vi "e.gate HighSpeedPort Query.vi"(0 "TCP-Connection (Refnum in)":refnum<k5>, 5 "Command (In)":string, 7 "Timeout":i32, 9 "TCP LengthRead":i32, 11 "error in (no error)":errorcluster) -> (4 "TCP-Connection (Refnum out)":refnum<k5>, 6 "Data (out - binary)":u8[](array[numeric]), 8 "data out (string)":string, 15 "error out":errorcluster)   [LabVIEW 2016]
doc: "This VI is used for data transfer over HighSpeedPort TCP/IP."
panel:
  out "Daten":string
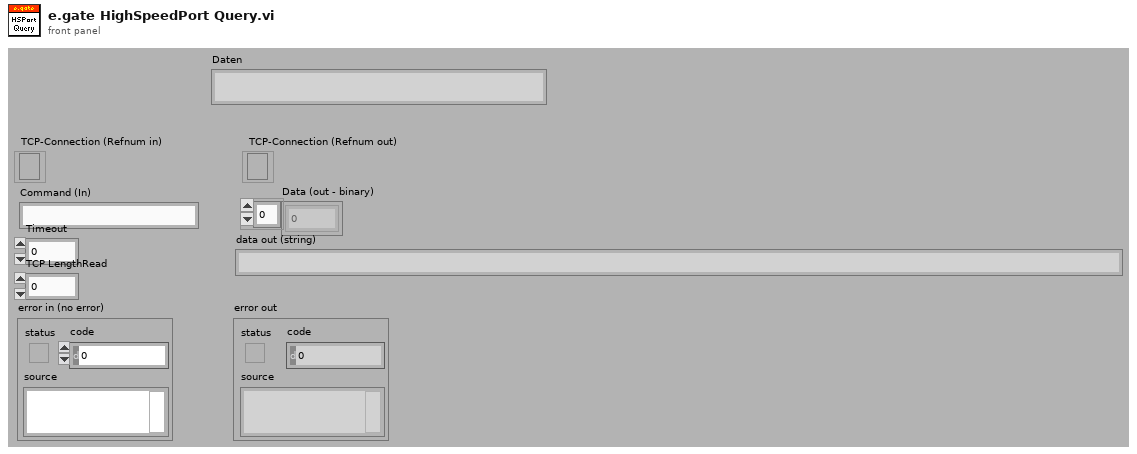
[diagram p1: front panel]
types:
  T1 = enum16{"Standard", "Buffered", "CRLF", "Immediate"}
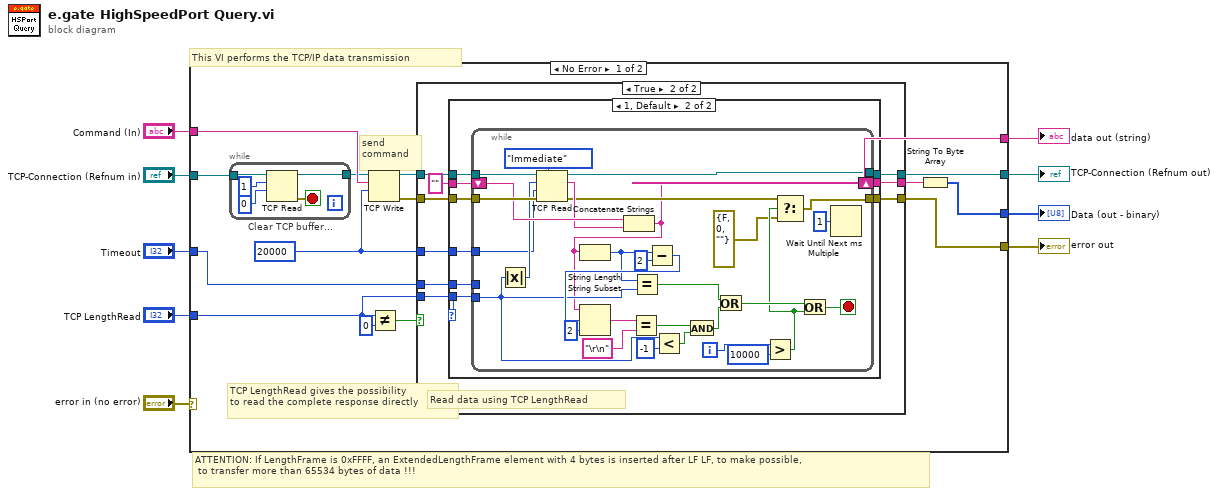
[diagram p0: block diagram]
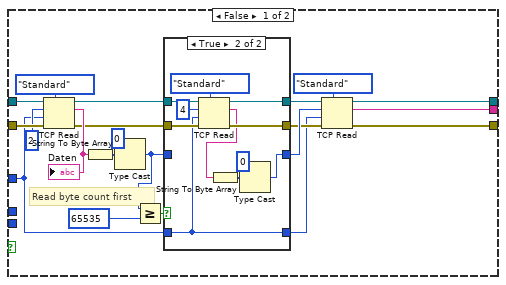
[diagram p2: hidden frame]
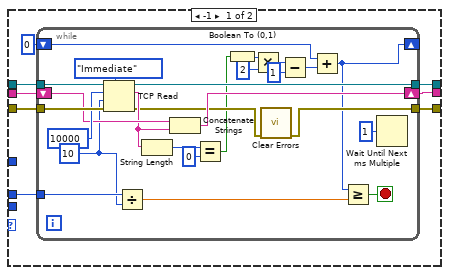
[diagram p4: hidden frame]
diagram:
  # "ATTENTION: If LengthFrame is 0xFFFF, an ExtendedLengthFrame element with 4 bytes is inserted after LF LF, to make possible,\n\tto transfer more than 65534 bytes of data !!!"
  # "This VI performs the TCP/IP data transmission"
  n1 = case shown="No Error" "error in (no error)" {
    selector: "error in (no error)" -> [_ w146]
    tunnel: "TCP-Connection (Refnum in)" -> [w20 w147]
    tunnel: "Timeout" -> [w11 _]
    tunnel: [w23 w147] -> w7
    tunnel: [w22 w146] -> w1
    tunnel: [w21 _] -> w6
    tunnel: "TCP LengthRead" -> [w19 _]
    tunnel: [w18 _] -> w4
    tunnel: "Command (In)" -> [w17 _]
    frame No Error {
      w10 = 20000 ("Timeout")
      # "TCP LengthRead gives the possibility\nto read the complete response directly"
      # "send\ncommand"
      n2 = while "Clear TCP buffer..." {
        tunnel: [w144] -> w14
        tunnel: w20 -> [w141]
        stop <- w145 stop-if-true
        n3 = TCP Read(connection ID=w141, bytes to read=1, 9:0 ("Timeout in ms (25000)")) -> (connection ID out=w144:refnum<k5>, error out=w145:errorcluster)  [unwired: 1 in, 2 out]
      }
      n4 = TCP Write ("TCP: Schreiben")(connection ID=w14, data in=w17, 9:w10) -> (connection ID out=w15:refnum<k5>, error out=w16:errorcluster)  [unwired: 1 in, 1 out]
      n5 = Not Equal?(x=w19, y=0) -> (x != y?=w12:bool)
      n6 = case shown="True" w12 {
        tunnel: w16 -> [w44 w67]
        tunnel: w15 -> [w43 w68]
        tunnel: [w36 w65] -> w23
        tunnel: [w35 w66] -> w22
        tunnel: [w34 w64] -> w18
        tunnel: w10 -> [w25 w63]
        tunnel: w19 -> [_ w60]
        tunnel: w11 -> [_ w61]
        frame False {
          # "Read byte count first"
          n7 = TCP Read ("TCP: Lesen")(connection ID=w43, bytes to read=2 ("Bytes zu lesen"), error in (no error)=w44, 7:T1."Standard" ("Modus (Standard)"), 9:w25) -> (connection ID out=w30:refnum<k5>, data out=w38:string, error out=w32:errorcluster)
          "Daten" <- w38
          n8 = String To Byte Array(string=w38) -> (unsigned byte array=w39:u8[])
          n9 = Type Cast(type=u16 0, x=w39) -> (*(type *) &x=w27:u16)
          n10 = Greater Or Equal?(x=w27, y=65535) -> (x >= y?=w28:bool)
          n11 = case shown="True" w28 {
            tunnel: w27 -> [w48 _]
            tunnel: [w48 w49] -> w33
            tunnel: w32 -> [w47 w56]
            tunnel: [w47 w55] -> w31
            tunnel: w30 -> [w46 w57]
            tunnel: [w46 w58] -> w29
            tunnel: w25 -> [w45 w54]
            tunnel: [w45 w54] -> w24
            frame False {
            }
            frame True {
              n12 = TCP Read ("TCP: Lesen")(connection ID=w57, bytes to read=4 ("Bytes zu lesen"), error in (no error)=w56, 7:T1."Standard" ("Modus (Standard)"), 9:w54) -> (connection ID out=w58:refnum<k5>, data out=w50:string, error out=w55:errorcluster)
              n13 = String To Byte Array(string=w50) -> (unsigned byte array=w52:u8[])
              n14 = Type Cast(type=u32 0, x=w52) -> (*(type *) &x=w49:u32)
            }
          }
          n15 = TCP Read ("TCP: Lesen")(connection ID=w29, bytes to read=w33, error in (no error)=w31, 7:T1."Standard" ("Modus (Standard)"), 9:w24) -> (connection ID out=w36:refnum<k5>, data out=w34:string, error out=w35:errorcluster)
        }
        frame True {
          # "Read data using TCP LengthRead"
          n16 = case shown="1, Default" w60 {
            tunnel: w68 -> [w73 w110]
            tunnel: w67 -> [w71 w109]
            tunnel: [w74 w108] -> w66
            tunnel: [w75 w107] -> w65
            tunnel: [w76 w106] -> w64
            tunnel: w63 -> [_ w105]
            tunnel: w60 -> [_ w104]
            tunnel: "" -> [w72 w103]
            tunnel: w61 -> [w70 w102]
            frame -1 {
              n17 = while {
                tunnel: w73 -> [w101]
                tunnel: [w99] -> w75
                shift-right: [w94] -> w76
                shift-left: w72 -> [w95]
                tunnel: w71 -> [w100]
                tunnel: [w85] -> w74
                tunnel: w70 -> [w90]
                shift-right: [w77] -> _
                shift-left: 0 ("y") -> [w91]
                stop <- w87 stop-if-true
                w89 = 10 ("Timeout in ms (25000)")
                n18 = TCP Read(connection ID=w101, bytes to read=10000 ("Bytes zu lesen"), error in (no error)=w100, 7:T1."Immediate" ("Modus (Standard)"), 9:w89) -> (connection ID out=w99:refnum<k5>, data out=w92:string, error out=w86:errorcluster)
                n19 = Divide(x=w90, y=w89) -> (x/y=w88:dbl)
                n20 = String Length(string=w92) -> (length=w84:i32)
                n21 = Concatenate Strings(w95, w92) -> (w94:string)
                n22 = Equal?(x=w84, y=0) -> (x = y?=w83:bool)
                n23 = Boolean To (0,1)(Boolean=w83) -> (0, 1=w82:i16)
                n24 = Multiply(x=w82, y=i16 2) -> (x*y=w80:i16)
                n25 = call <vilib>:"Clear Errors.vi"("error in (no error)"=w86) -> ("error out"=w85:errorcluster)  [unwired: 1 in, 5 out]
                n26 = Subtract(x=w80, y=i16 1) -> (x-y=w78:i16)
                n27 = Add(x=w91, y=w78) -> (x+y=w77:i32)
                n28 = Greater Or Equal?(x=w77, y=w88) -> (x >= y?=w87:bool)
                n29 = Wait Until Next ms Multiple(millisecond multiple=u32 1 ("Vielfache von ms")) -> ()  [unwired: 1 out]
              }
            }
            frame 1, Default {
              n30 = while {
                tunnel: w110 -> [w140]
                tunnel: [w138] -> w107
                tunnel: w105 -> [w113]
                tunnel: w104 -> [w124]
                shift-right: [w111] -> w106
                shift-left: w103 -> [w136]
                tunnel: w102 -> [_]
                tunnel: w109 -> [w139]
                tunnel: [w117] -> w108
                i -> [w120]
                stop <- w112 stop-if-true
                n31 = Absolute Value(x=w124) -> (abs(x)=w123:i32)
                n32 = TCP Read(connection ID=w140, bytes to read=w123, error in (no error)=w139, 7:T1."Immediate" ("Modus (Standard)"), 9:w113) -> (connection ID out=w138:refnum<k5>, data out=w135:string, error out=w116:errorcluster)
                n33 = Concatenate Strings(w136, w135) -> (w111:string)
                n34 = String Length(string=w111) -> (length=w114:i32)
                n35 = Equal?(x=w114, y=w124) -> (x = y?=w125:bool)
                n36 = Subtract(x=w114, y=2) -> (x-y=w133:i32)
                n37 = String Subset(string=w111, offset (0)=w133, length (rest)=2 ("Länge (Rest)")) -> (substring=w131:string)
                n38 = Equal?(x=w131, y="\r\n") -> (x = y?=w129:bool)
                n39 = Less?(x=w124, y=-1) -> (x < y?=w128:bool)
                n40 = And(x=w129, y=w128) -> (x .and. y?=w126:bool)
                n41 = Or(x=w125, y=w126) -> (x .or. y?=w121:bool)
                n42 = Greater?(x=w120, y=10000) -> (0:w118:bool)
                n43 = Select(t=w116, s=w118, f=errorcluster {"status"=FALSE, "code"=0, "source"=""}) -> (s? t:f=w117:errorcluster)
                n44 = Or(x=w121, y=w118) -> (x .or. y?=w112:bool)
                n45 = Wait Until Next ms Multiple(millisecond multiple=u32 1 ("Vielfache von ms")) -> ()  [unwired: 1 out]
              }
            }
          }
        }
      }
      n46 = String To Byte Array(string=w18) -> (unsigned byte array=w21:u8[])
    }
    frame Error {
    }
  }
  "TCP-Connection (Refnum out)" <- w7
  "Data (out - binary)" <- w6
  "data out (string)" <- w4
  "error out" <- w1
